vi "ex4-7.vi"() -> ()   [LabVIEW 2009]
uses:
  <vilib>/NXT/Dual Mode Library/Waits/Wait_Num.vi
  <vilib>/NXT/Dual Mode Library/Motors/MotorReverse.vi
  <vilib>/NXT/Dual Mode Library/Motors/MotorOn.vi
panel:
  in  "Y":dbl
  in  "X":dbl
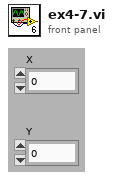
[diagram p1: front panel]
types:
  T1 = typedef "LVHSConnector.ctl" = cluster{"error":errorcluster, "address":string, "NXT #":i32, "Show Error":bool, "Connection":u16}
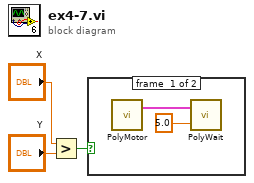
[diagram p0: block diagram]
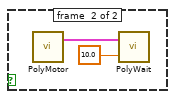
[diagram p2: hidden frame]
diagram:
  n1 = Greater?(x="X", y="Y") -> (0:w1:bool)
  n2 = case shown="False" w1 {
    frame #0 {
      n3 = call-poly <vilib>:"PolyMotor.vi"() -> ("NXT"=w5:T1)  [unwired: 4 in]
      n4 = call-poly <vilib>:"PolyWait.vi"("Time (1 sec)"=sgl 5.0, "NXT"=w5) -> ()  [unwired: 2 in, 1 out]
    }
    frame #1 {
      n5 = call-poly <vilib>:"PolyMotor.vi"() -> ("NXT"=w7:T1)  [unwired: 4 in]
      n6 = call-poly <vilib>:"PolyWait.vi"("Time (1 sec)"=sgl 10.0, "NXT"=w7) -> ()  [unwired: 2 in, 1 out]
    }
  }
